vi "Avantes - AVS_Activate.vi"(8 "error in (no error)":errorcluster, 11 "AVS Settings In":T1) -> (0 "error out":errorcluster, 3 "AVS Settings Out":T1)   [LabVIEW 2014, in "AvaSpec.lvlib" / "Avantes Spectrometer Functions.lvlib"]
uses:
  Avantes Spectrometer Functions.lvlib
  AVS settings.ctl
  AvaSpec.lvlib
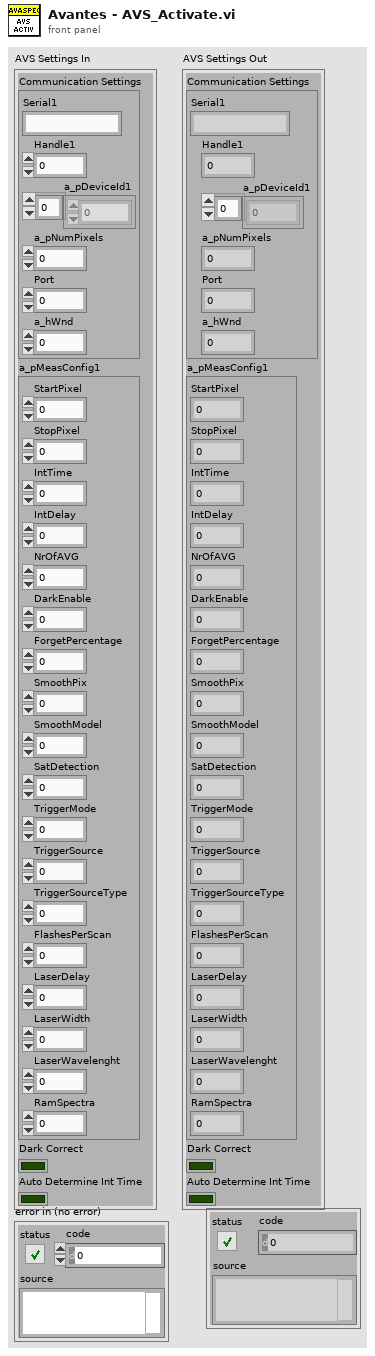
[diagram p1: front panel]
types:
  T1 = typedef "AvaSpec.lvlib/AVS settings.ctl" = cluster{"Communication Settings":cluster{"Serial1":string, "Handle1":i32, "a_pDeviceId1":u8[], "a_pNumPixels":u16, "Port":i32, "a_hWnd":i32}, "a_pMeasConfig1":cluster{"StartPixel":u16, "StopPixel":u16, "IntTime":sgl, "IntDelay":u32, "NrOfAVG":u32, "DarkEnable":u8, "ForgetPercentage":u8, "SmoothPix":u16, "SmoothModel":u8, "SatDetection":u8, "TriggerMode":u8, "TriggerSource":u8, "TriggerSourceType":u8, "FlashesPerScan":u16, "LaserDelay":u32, "LaserWidth":u32, "LaserWavelenght":sgl, "RamSpectra":u16}, "Dark Correct":bool, "Auto Determine Int Time":bool}
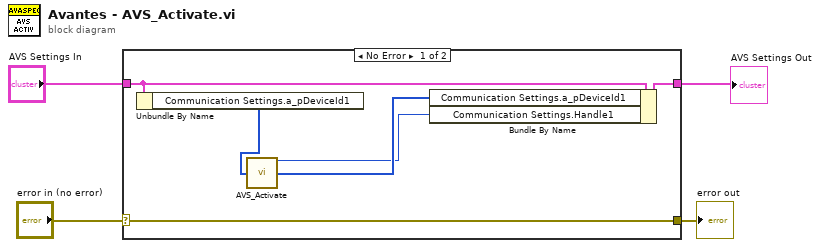
[diagram p0: block diagram]
diagram:
  n1 = case shown="No Error" "error in (no error)" {
    selector: "error in (no error)" -> [w10 w12]
    tunnel: [w9 w11] -> w1
    tunnel: "AVS Settings In" -> [w6 w11]
    tunnel: [w10 w12] -> w3
    frame No Error {
      n2 = Unbundle By Name(w6) -> ("Communication Settings.a_pDeviceId1"=w5:u8[])
      n3 = call "AVS_Activate.vi"("a_pDeviceId"=w5) -> ("Output Value"=w7:i32, "a_pDeviceId"=w8:u8[])  [unwired: 13 in]
      n4 = Bundle By Name(cluster=w6, "Communication Settings.a_pDeviceId1"=w8, "Communication Settings.Handle1"=w7) -> (w9:T1)
    }
    frame Error {
    }
  }
  "error out" <- w3
  "AVS Settings Out" <- w1
